vi "Status Bar.vi"() -> ()   [LabVIEW 2012]
panel:
  in  "ImageList":refnum<k7>(container)
  in  "status text":string
  in  "Stop":bool
  in  "StatusBar":refnum<k7>(container)
  # "Using the Microsoft StatusBar Control (6.0) in LabVIEW"
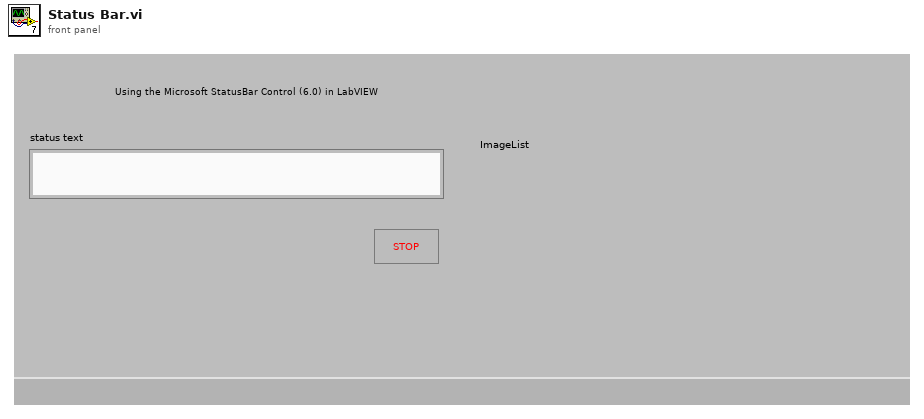
[diagram p1: front panel]
types:
  T1 = enum16{"Sticks Top/Left", "Sticks Bottom/Right", "Proportional"}
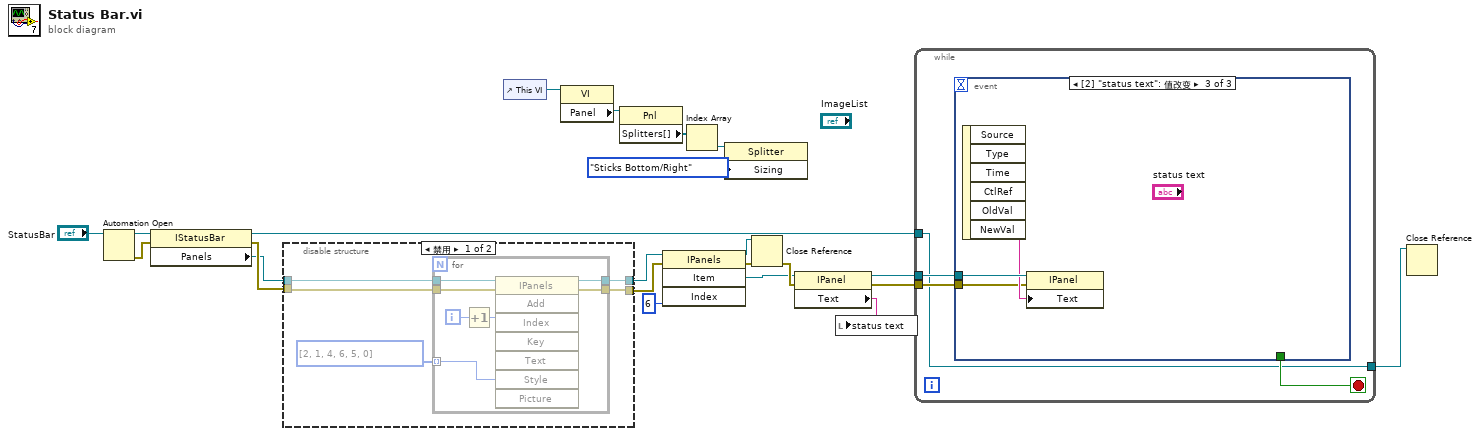
[diagram p0: block diagram]
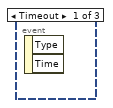
[diagram p3: hidden frame]
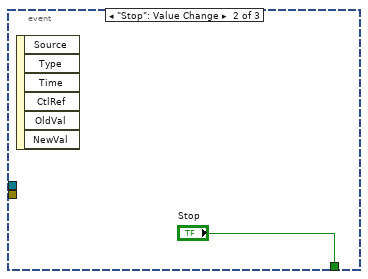
[diagram p4: hidden frame]
diagram:
  n1 = Automation Open(Automation Refnum="StatusBar") -> (Automation Refnum=w20:refnum<k7>, error out=w19:errorcluster)  [unwired: 1 in, 2 out]
  n2 = property class="IStatusBar"(reference=w20, error in=w19) -> (reference out=w7:refnum<k7>, error out=w4:errorcluster, "Panels"=w3:refnum<k7>)
  n3 = disable-structure shown="禁用" {
    disable-tunnel: w3 -> [w26 w36]
    disable-tunnel: w4 -> [w25 w35]
    disable-tunnel: [w24 w36] -> w2
    disable-tunnel: [w23 w35] -> w1
    frame Disabled {
      w27 = i32[] [2, 1, 4, 6, 5, 0] items=["sbrText", "sbrCaps", "sbrNum", "sbrIns", "sbrScrl", "sbrTime", "sbrDate", "sbrKana"]
      n4 = for {
        tunnel: w26 -> [w34]
        tunnel: w25 -> [w33]
        tunnel: w27 -> [w32] mode=indexing
        tunnel: [w29] -> w23
        tunnel: [w28] -> w24
        i -> [w31]
        n5 = Increment(x=w31) -> (x+1=w30:i32)
        n6 = invoke class="IPanels" method="Add"(reference=w34, error in=w33, "Index"=w30, "Style"=w32) -> (reference out=w28:refnum<k7>, error out=w29:errorcluster)  [unwired: 4 in, 6 out]
      }
    }
    frame Enabled {
    }
  }
  n7 = control-ref of="This VI"() -> (w22:refnum<vi>)
  n8 = property class="VI"(reference=w22) -> ("Panel"=w21:refnum<vi>)  [unwired: 1 in, 2 out]
  n9 = property class="Pnl"(reference=w21) -> ("Splitters[]"=w10:refnum<vi>[])  [unwired: 1 in, 2 out]
  n10 = invoke class="IPanels" method="Item"(reference=w2, error in=w1, "Index"=6) -> (reference out=w15:refnum<k7>, error out=w14:errorcluster, "Item"=w8:refnum<k7>)  [unwired: 1 in, 1 out]
  n11 = Index Array(array=w10) -> (element=w9:refnum<vi>)  [unwired: 1 in]
  n12 = property class="Splitter"(reference=w9, "Sizing"=T1."Sticks Bottom/Right") -> ()  [unwired: 1 in, 2 out]
  n13 = Close Reference(reference=w15, error in (no error)=w14) -> (error out=w13:errorcluster)
  n14 = property class="IPanel"(reference=w8, error in=w13) -> (reference out=w16:refnum<k7>, error out=w6:errorcluster, "Text"=w17:string)
  n15 = local write "status text"(w17) -> ()
  n16 = while {
    tunnel: w16 -> [w39]
    tunnel: w7 -> [w37]
    tunnel: w6 -> [w38]
    tunnel: [w37] -> w12
    stop <- w40 stop-if-true
    n17 = event shown="[2] \"status text\": 值改变" {
      selector: _ -> [_ _ _]
      dyn-events: _ -> [_ _ _]
      timeout: _ -> [_ _ _]
      tunnel: [_ "Stop" _] -> w40
      tunnel: w39 -> [_ _ w44]
      tunnel: w38 -> [_ _ w42]
      event Timeout {
        n18 = event-data() -> ()  [unwired: 3 out]
      }
      event "Stop": Value Change {
        n19 = event-data() -> ()  [unwired: 7 out]
      }
      event "status text": Value Change {
        n20 = event-data() -> ("NewVal"=w43:string)  [unwired: 6 out]
        n21 = property class="IPanel"(reference=w44, error in=w42, "Text"=w43) -> ()  [unwired: 2 out]
      }
    }
  }
  n22 = Close Reference(reference=w12) -> ()  [unwired: 1 in, 1 out]
